vi "Dashboard Main.vi"() -> ()   [LabVIEW 2014]
uses:
  robot/Lightning base/Auton Modes.ctl
  <vilib>/event_ctls.llb/eventvkey.ctl
  VideoControlMode.ctl
  Video State.vi
  <vilib>/Rock Robotics/WPI/Dashboard/WPI_DashboardLogging Global.vi
  <vilib>/Utility/config.llb/Write Key (String).vi
  <vilib>/Utility/config.llb/Write Key (I32).vi
  <vilib>/Rock Robotics/Network Tables/SD Write Number.vi
  <vilib>/Utility/config.llb/NI_LVConfig.lvlib
panel:
  out "Video Mode":bool
  out "OpenIniState":enum16{"Waiting", "SwitchModeHappening"}(ring)
  out "Joystick":dbl
  out "POV[0]":dbl
  out "CameraSwitchModeState":enum16{"Waiting", "SwitchModeHappening"}(ring)
  out "Camera Mode":bool
  out "GetIniState":enum16{"Waiting", "SwitchModeHappening"}(ring)
  out "SetIniState":enum16{"Waiting", "SwitchModeHappening"}(ring)
  in  "TCP":refnum<k5>
  in  "Rec Mode":enum32{"Stop", "Record", "Playback"}(radio)
  in  "Vision":u16(ring) items=["Camera Off", "USB Camera SW", "USB Camera HW", "IP Camera"]
  out "Camera IP":string
  out "Image Message":string="Timeout in Camera Communications"
  in  "Dashboard Tab":T1(tab)=enum."Auton"
  in  "Camera Settings":T2={"Frame Rate"=30, "Compression"=30, "Size"=1} {"Frame Rate" scale=1.0..30.0; "Size" items=["640x480", "320x240", "160x120"]}
  out "MotorChart R":cluster{"Numeric":dbl, "Numeric":dbl}(graph)
  out "MotorChart L":T3(graph)
  out "MotorSliders R":cluster{"MotorSlide1":dbl, "MotorSlide2":dbl} {"MotorSlide2" scale=-1.0..1.0 scale format="%#_2e"; "MotorSlide1" scale=-1.0..1.0 scale format="%#_2e"}
  out "MotorSliders L":T4 {"MotorSlide4 2" scale=0.0..14.0 scale format="%#_2e"; "MotorSlide2" scale=-1.0..1.0 scale format="%#_2e"; "MotorSlide1" scale=-1.0..1.0 scale format="%#_2e"}
  out "Gyro":dbl(knob) scale=0.0..360.0
  out "JS1 Z":dbl(slide) scale=-1.0..1.0 scale format="%#_2e"
  out "JS1 Graph":cluster{"X":dbl, "Y":dbl}[](graph)
  out "JS1 Buttons":T5
  out "JS2 Z":dbl(slide) scale=-1.0..1.0 scale format="%#_2e"
  out "JS2 Graph":cluster{"X":dbl, "Y":dbl}[](graph)
  out "JS2 Buttons":T5
  out "Mode":T6(ring)=enum."Auto Disabled"
  in  "DB Camera Config":bool
  out "fps":dbl format="%#.1g"
  out "Mbps":dbl format="%#.1g"
  out "Mbps 2":bool
  in  "Camera Joystick Controller":enum16{"Joystick 1", "Joystick 2"}(ring)
  in  "Camera Choice":enum16{"Front", "Back"}(ring)
  in  "CG Drive Delay":dbl
  in  "CG Power2":dbl
  in  "CG Drive Distance":dbl
  in  "CG Power":dbl
  in  "CG Time2":dbl
  in  "CG Time":dbl
  in  "DriverAutonFile":string
  in  "CoPilotAutonFile":string
  in  "Auton Distance":dbl=2.0
  in  "Auton Mode":T7
  out "FTP Result":u32(colorbox)
  in  "Open INI File":bool
  in  "RoboRIO IP address":string="10.8.62.12"
  in  "Robot Full Path":string="/home/lvuser/calibrations/cals.ini"
  in  "Local Path":path=path "C:/FRC/Calibrations/cals.ini"
  in  "Send INI":bool
  in  "Get INI File":bool
  in  "Test Slider":dbl(slide) scale=0.0..100.0 scale format="%#_3g"
  in  "On/Off":bool caption="Solenoid"
  in  "Test Name":u16(ring) items=["Select the test to run...", "Example Test", "-------------------------------", "List of tests is built in robot code.", "Replace with your own automated tests."]
  in  "Test Tree":string(tree)
  in  "Motor":cluster{"Value":dbl, "Enable":bool} {"Value" scale=-1.0..1.0 scale format="%#_3g"}
  out "Progress":T8 {"Test Progress" scale=0.0..100.0}
  in  "Rev/Fwd":cluster{"Forward":bool, "Reverse":bool}
  in  "Test Ring":u16(ring) items=["Monochrome", "Color"]
  in  "Listbox":i32(listbox)
  out "Tree":string(tree)
  in  "PID":bool
  in  "DeadZone":dbl
  in  "PIDi":dbl
  in  "PIDd":dbl
  in  "Max Velocity":dbl
  in  "DriveRamp":dbl
  in  "PIDp":dbl
  in  "DriveSkew":dbl
  in  "MinMotorPower":dbl
  in  "MinJoystickChange":dbl
  in  "Drive Slice Time":dbl
  out "Camera Image":T9(plugin-control)
  out "Boolean":bool
  # "Left"
  # "Front"
  # "Right"
  # "Battery"
  # "Base file names, assumed to be\n/home/lvuser/auton"
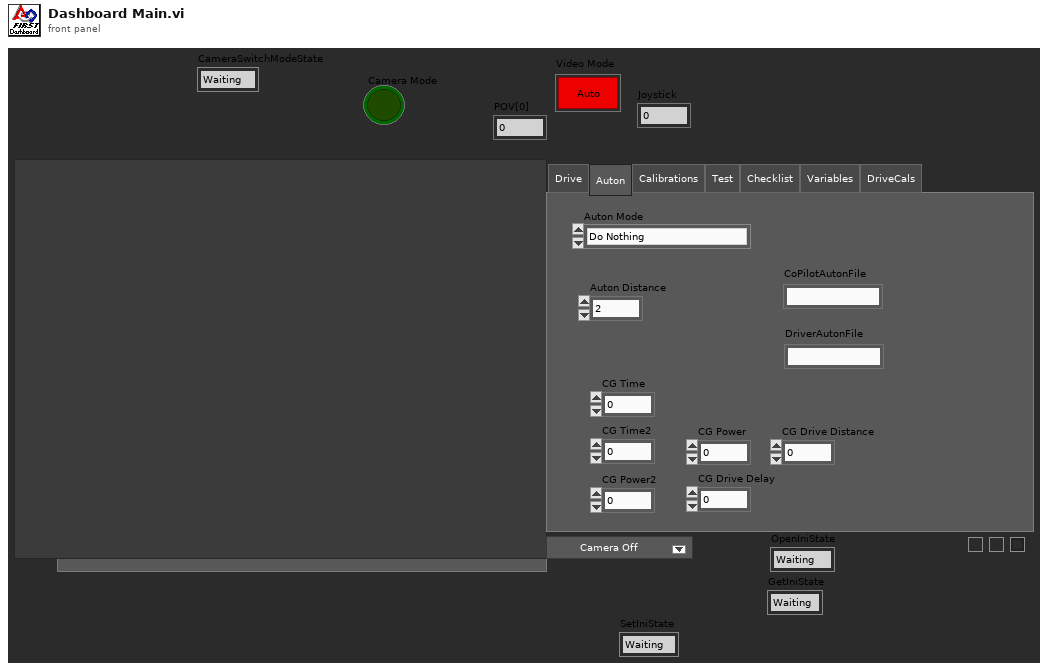
[diagram p1: front panel]
types:
  T1 = enum32{"Drive", "Auton", "Calibrations", "Test", "Checklist", "Variables", "DriveCals"}
  T2 = cluster{"Frame Rate":i32, "Compression":i32, "Size":u16}
  T3 = cluster{"Numeric":dbl, "Numeric":dbl, "Battery V":dbl}
  T4 = cluster{"MotorSlide1":dbl, "MotorSlide2":dbl, "MotorSlide4 2":dbl}
  T5 = cluster{bool, bool, bool, bool, bool, bool, bool, bool, bool, bool, bool, bool}
  T6 = enum8{"Tele-Op Disabled", "Tele-Op Enabled", "Auto Disabled", "Auto Enabled", "Test Disabled", "Test Enabled", "Disconnected", "No Code", "E-Stop"}
  T7 = typedef "Auton Modes.ctl" = enum16{"Do Nothing", "Snake", "Move Forward", "Move Forward w/Tote", "Move Forward w/RC", "Gather RC from Step", "3 Tote Auton", "Vision Test", "Strafer", "Pick up rc"}
  T8 = cluster{"Test Progress":u8, "Test Progress Text":string}
  T9 = typedef "IMAQ Image.ctl" = refnum<image>
  T10 = enum32{"Drive", "Basic", "Custom", "Test", "Checklist", "Variables", "DriveCals"}
  T11 = enum32{"Drive", "Basic", "Custom", "Test", "Checklist", "Variables"}
  T12 = enum32{"Drive", "Auton", "Custom", "Test", "Checklist", "Variables"}
  T13 = typedef "Image Type" = u32
  T14 = enum16{"Waiting", "SwitchModeHappening", "SwitchDone"}
  T15 = typedef "VideoControlMode.ctl" = enum16{"HatControl", "JoystickControl"}
  T16 = cluster{"Camera Image":refnum<vi>, "Dashboard Tab":refnum<vi>, "Boolean":refnum<vi>, "Vision":refnum<vi>, "Rec Mode":refnum<vi>, "Test Slider":refnum<vi>, "On/Off ":refnum<vi>, "Test Ring":refnum<vi>, "Rev/Fwd":refnum<vi>, "Test Name":refnum<vi>, "Motor":refnum<vi>, "Progress":refnum<vi>, "CheckList":refnum<vi>, "Tree":refnum<vi>, "Test Tree":refnum<vi>}
  T17 = cluster{"Desired Font (Application)":enum16{"User-specified Font", "Application Font", "System Font", "Dialog Font"}, "[User-specified Font]":cluster{"Font Name":string, "Size":i16, "Strikeout?":bool, "Italic?":bool, "Underline?":bool, "Outline?":bool, "Shadow?":bool, "Bold?":bool, "Rotation Angle":dbl}, "Horizontal Alignment":i16, "Vertical Alignment":i16}
  T18 = cluster{"Error Strings":string, "Disable Counts":cluster{u16, u16}, "Rail Faults":cluster{u16, u16, u16}, "Robot IP":string, "DB Mode":u8, "Event Info":cluster{"Name":string, "Type":u8, "Number":u16, "Replay":u8}, "Camera Addr":string}
  T19 = cluster{"Storage":cluster{"Disk Free":u64, "RAM Block":u32, "RAM free":u32}, "CPU Utilization":cluster{"CPU % ISR":sgl, "CPU % Time Crit":sgl, "CPU % Timed Str":sgl, "CPU % High":sgl, "CPU % Above":sgl, "CPU % Normal":sgl, "CPU % Low":sgl}, "CAN":cluster{"% Bus Utilization":sgl, "Bus Off Cnt":u32, "TX_FIFO Full Cnt":u32, "Receive Error Cnt":u8, "Transmit Error Cnt":u8}, "HID":cluster{"HID Outputs":u32, "Rumble Low":u16, "Rumble High":u16}[]}
  T20 = cluster{"Status bits":cluster{"Test Mode":bool, "Autonomous":bool, "Enabled":bool, "Code Start":bool, "Brownout":bool, "Reserved 2":bool, "Reserved 3":bool, "E-Stop":bool}, "Code Trace":cluster{"Disabled":bool, "TeleOp":bool, "Auto":bool, "Test":bool}, "Controller Type":enum16{"unknown", "cRIO", "roboRio"}, "Code?":enum16{"unknown", "noCode", "code"}, "Battery V":dbl}
  T21 = cluster{"Control Bits":cluster{"TestMode":bool, "Autonomous":bool, "Enabled":bool, "FMS Present":bool, bool, bool, bool, "E-Stop":bool}, "Team Station ":u8, "Countdown":sgl, "Joystick Values":cluster{"Axes":dbl[], "Buttons":bool[], "POVs":i16[]}[]}
  T22 = cluster{"Axes":dbl[], "Buttons":bool[], "POVs":i16[]}[]
  T23 = cluster{"Disabled":bool, "TeleOp":bool, "Auto":bool, "Test":bool}
  T24 = cluster{"Axes":dbl[], "Buttons":bool[], "POVs":i16[]}
  T25 = cluster{"Buttons[0]":bool, "Buttons[1]":bool, "Buttons[2]":bool, "Buttons[3]":bool, "Buttons[4]":bool, "Buttons[5]":bool, "Buttons[6]":bool, "Buttons[7]":bool, "Buttons[8]":bool}
  T26 = cluster{"POVs[0]":i16, "POVs[1]":i16, "POVs[2]":i16, "POVs[3]":i16, "POVs[4]":i16, "POVs[5]":i16, "POVs[6]":i16, "POVs[7]":i16, "POVs[8]":i16}
  T27 = cluster{"Axes[0]":dbl, "Axes[1]":dbl, "Axes[2]":dbl, "Axes[3]":dbl, "Axes[4]":dbl, "Axes[5]":dbl, "Axes[6]":dbl, "Axes[7]":dbl, "Axes[8]":dbl}
  T28 = cluster{"Buttons[0]":bool, "Buttons[1]":bool, "Buttons[2]":bool, "Buttons[3]":bool, "Buttons[4]":bool, "Buttons[5]":bool, "Buttons[6]":bool, "Buttons[7]":bool, "Buttons[8]":bool, "Buttons[9]":bool, "Buttons[10]":bool, "Buttons[11]":bool}
  T29 = typedef "NI_LVConfig.lvlib/Config Data RefNum.ctl" = refnum<k1>
  T30 = cluster{"Operation":enum16{"Update", "Clear"}, "Color Box":u32}[]
  T31 = typedef "eventvkey.ctl" = enum16{"ASCII", "Enter", "Return", "Shift", "Ctrl", "Alt", "Cmd", "Opt", "Caps", "NumLock", "Clear", "Break", "Up", "Down", "Left", "Right", "Insert", "Delete", "Home", "End", "PageUp", "PageDown", "Escape", "Help", "Pause", "ScrollLock", "F1", "F2", "F3", "F4", "F5", "F6", "F7", "F8", "F9", "F10", "F11", "F12", "F13", "F14", "F15", "F16", "F17", "F18", "F19", "F20", "F21", "F22", "F23", "F24", "Play", "VolumeUp", "VolumeDown", "Mute", "Two Byte Char"}
  T32 = cluster{"Image Size":bool, "Image Type":bool, "Pixel Value":bool, "ROI Information":bool, "Zoom Factor":bool}
  T33 = enum8{"Enabled", "Disabled", "Disabled and Grayed Out"}
  T34 = cluster{"Operation":enum16{"Update", "Clear"}, "Color Box":u32}
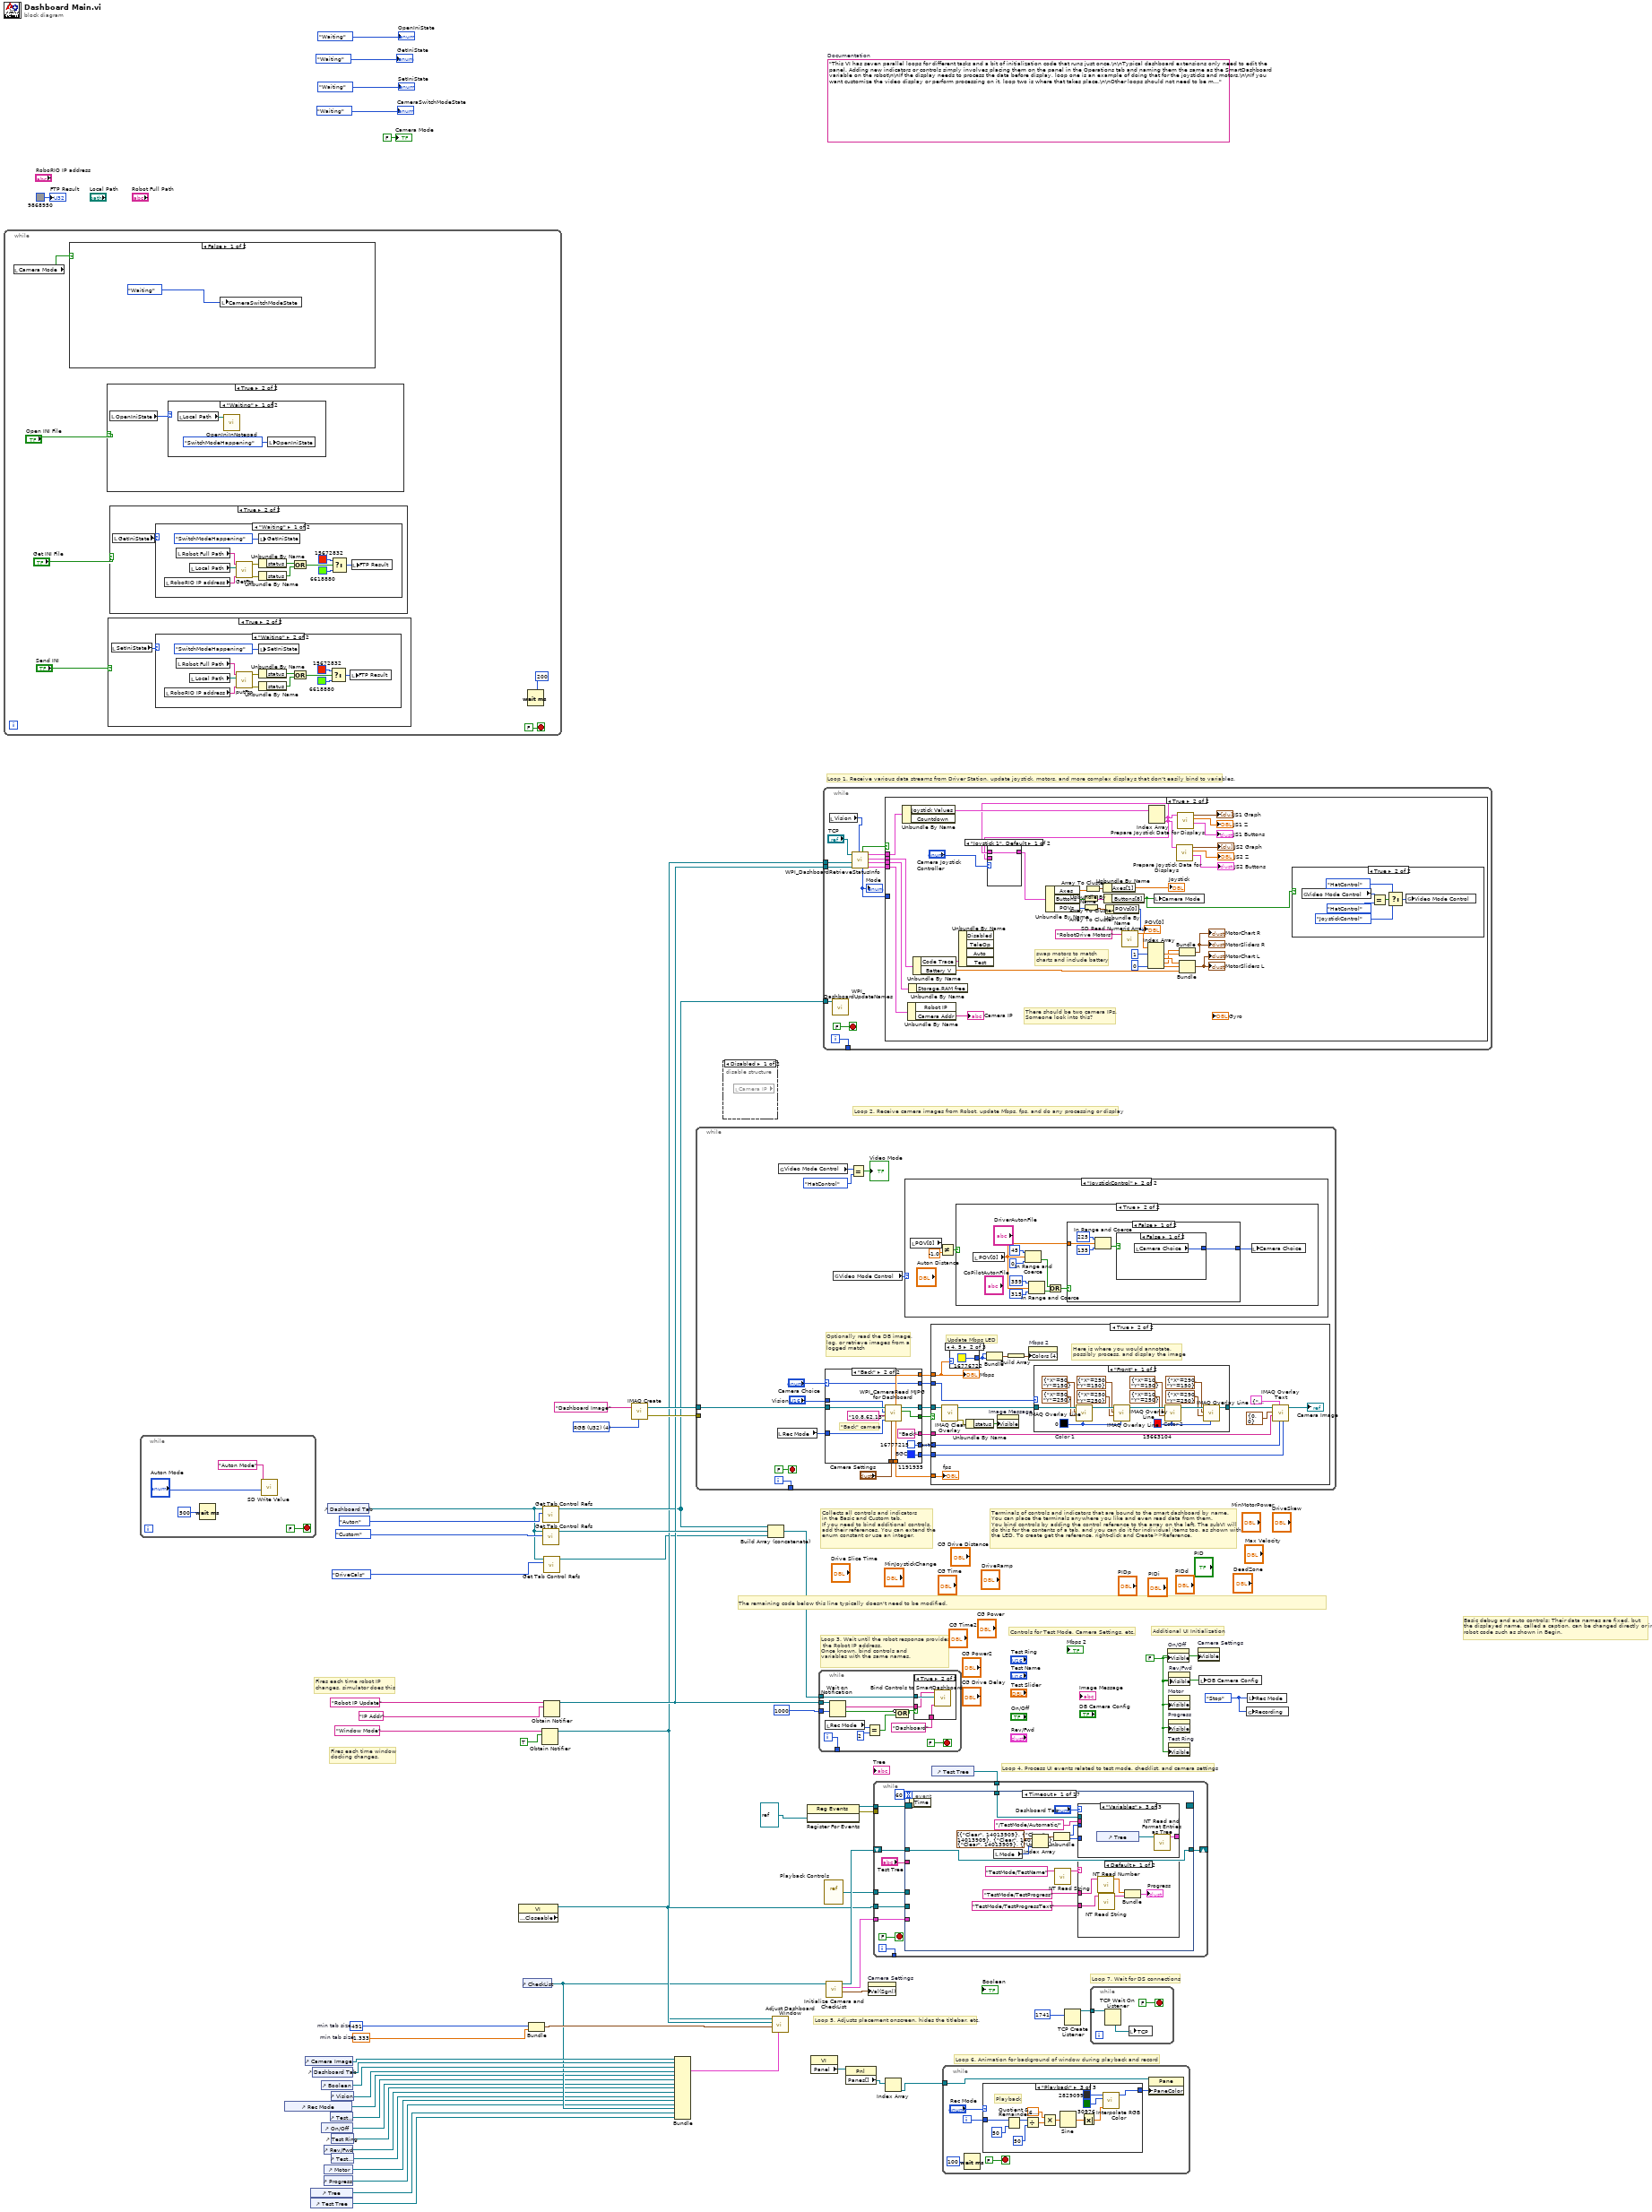
[diagram p0: block diagram]
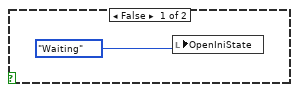
[diagram p3: hidden frame]
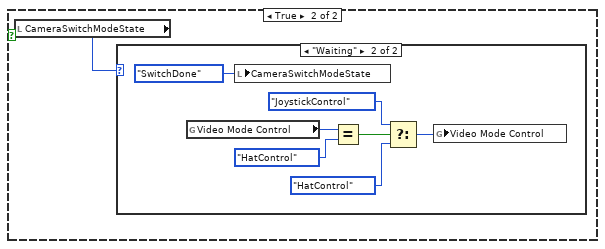
[diagram p5: hidden frame]
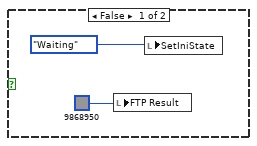
[diagram p7: hidden frame]
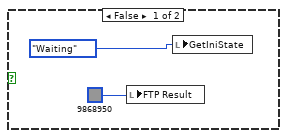
[diagram p9: hidden frame]
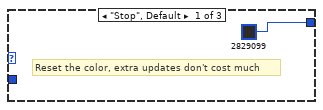
[diagram p14: hidden frame]
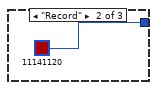
[diagram p15: hidden frame]
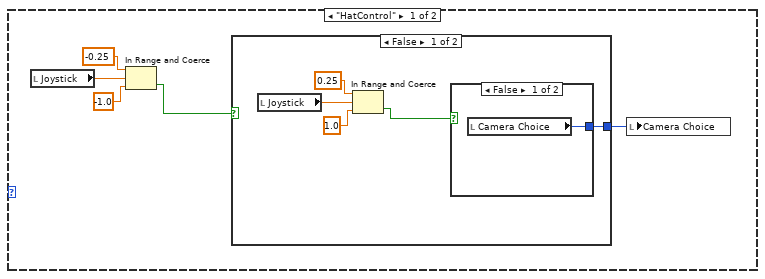
[diagram p17: hidden frame]
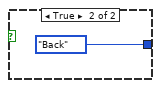
[diagram p18: hidden frame]
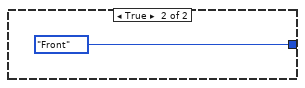
[diagram p19: hidden frame]
diagram:
  w33 = 491  # min tab size
  w32 = 1.333  # min tab size
  w40 = enum32{"Stop", "Record", "Playback"}."Stop" ("Rec Mode")
  w15 = FALSE ("Visible")
  (unwired) "This VI has seven parallel loops for different tasks and a bit of initialization code that runs just once.\n\nTypical dashboard extensions only need to edit the panel. Adding new indicators or controls simply involves placing them on the panel in the Operations tab and naming them the same as the SmartDashboard variable on the robot\n\nIf the display needs to process the data before display, loop one is an example of doing that for the joysticks and motors.\n\nIf you want customize the video display or perform processing on it, loop two is where that takes place.\n\nOther loops should not need to be modified. They are pretty standard, and document the task they perform."  # Documentation
  w60 = T13 4 items=["Grayscale (U8)", "Grayscale (I16)", "Grayscale (SGL)", "Complex (CSG)", "RGB (U32)", "HSL (U32)", "RGB (U64)"] ("Image Type")
  # "Loop 7. Wait for DS connections"
  # "Basic debug and auto controls: Their data names are fixed, but\nthe displayed name, called a caption, can be changed directly or in\nrobot code such as shown in Begin."
  # "Controls for Test Mode, Camera Settings, etc."
  # "Additional UI Initialization"
  # "Loop 6. Animation for background of window during playback and record"
  # "Fires each time robot IP\nchanges, simulator does this"
  # "Fires each time window\ndocking changes."
  # "Collects all controls and indicators\nin the Basic and Custom tab.\nIf you need to bind additional controls,\nadd their references. You can extend the\nenum constant or use an integer."
  # "The remaining code below this line typically doesn't need to be modified."
  # "Loop 4. Process UI events related to test mode, checklist, and camera settings"
  # "Terminals of controls and indicators that are bound to the smart dashboard by name.\nYou can place the terminals anywhere you like and even read data from them.\nYou bind controls by adding the control reference to the array on the left. The subVI will\ndo this for the contents of a tab, and you can do it for individual items too, as shown with\nthe LED. To create get the reference, right-click and Create>>Reference."
  # "Loop 3. Wait until the robot response provides\n the Robot IP address.\nOnce known, bind controls and\nvariables with the same names."
  # "Loop 5. Adjusts placement onscreen, hides the titlebar, etc."
  # "Loop 1. Receive various data streams from Driver Station, update joystick, motors, and more complex displays that don't easily bind to variables."
  # "Loop 2. Receive camera images from Robot, update Mbps, fps, and do any processing or display"
  n1 = while {
    stop <- FALSE stop-if-true
    n2 = local read "Camera Mode"() -> (w62:bool)
    n3 = case shown="False" w62 {
      frame False {
        n4 = local write "CameraSwitchModeState"(T14."Waiting" ("CameraSwitchMode")) -> ()
      }
      frame True {
        n5 = local read "CameraSwitchModeState"() -> (w72:enum16{"Waiting", "SwitchModeHappening"})
        n6 = case shown="\"Waiting\"" w72 {
          frame "SwitchModeHappening" {
          }
          frame "Waiting" {
            n7 = global read "Video State.vi" "Video Mode Control"() -> (w75:enum16{"HatControl", "JoystickControl"})
            n8 = local write "CameraSwitchModeState"(T14."SwitchDone" ("CameraSwitchMode")) -> ()
            n9 = Equal?(x=w75, y=enum16{"HatControl", "JoystickControl"}."HatControl" ("f")) -> (x = y?=w76:bool)
            n10 = Select(t=VideoControlMode."JoystickControl" ("f"), s=w76, f=enum16{"HatControl", "JoystickControl"}."HatControl") -> (s? t:f=w77:T15)
            n11 = global write "Video State.vi" "Video Mode Control"(w77) -> ()
          }
        }
      }
    }
    n12 = case shown="True" "Open INI File" {
      frame False {
        n13 = local write "OpenIniState"(T14."Waiting" ("GetIniState")) -> ()
      }
      frame True {
        n14 = local read "OpenIniState"() -> (w68:enum16{"Waiting", "SwitchModeHappening"})
        n15 = case shown="\"Waiting\"" w68 {
          frame "Waiting" {
            n16 = local read "Local Path"() -> (w69:path)
            n17 = call "OpenIniInNotepad.vi"("Path"=w69) -> ()  [unwired: 11 in]
            n18 = local write "OpenIniState"(T14."SwitchModeHappening" ("SetIniState")) -> ()
          }
          frame "SwitchModeHappening" {
          }
        }
      }
    }
    n19 = case shown="True" "Send INI" {
      frame False {
        n20 = local write "FTP Result"(u32 9868950 ("Color Box")) -> ()
        n21 = local write "SetIniState"(T14."Waiting" ("SetIniState")) -> ()
      }
      frame True {
        n22 = local read "SetIniState"() -> (w82:enum16{"Waiting", "SwitchModeHappening"})
        n23 = case shown="\"Waiting\"" w82 {
          frame "SwitchModeHappening" {
          }
          frame "Waiting" {
            n24 = local read "RoboRIO IP address"() -> (w93:string)
            n25 = local read "Robot Full Path"() -> (w92:string)
            n26 = local read "Local Path"() -> (w91:path)
            n27 = call "putFtp.vi"("host"=w93, "local path"=w91, "remote path"=w92) -> ("file error out"=w83:errorcluster, "ftp error out 2"=w84:errorcluster)  [unwired: 7 in]
            n28 = local write "SetIniState"(T14."SwitchModeHappening" ("SetIniState")) -> ()
            n29 = Unbundle By Name(w84) -> ("status"=w85:bool)
            n30 = Unbundle By Name(w83) -> ("status"=w86:bool)
            n31 = Or(x=w85, y=w86) -> (x .or. y?=w87:bool)
            n32 = Select(t=u32 15672832 ("Color Box"), s=w87, f=u32 6618880 ("Color Box")) -> (s? t:f=w88:u32)
            n33 = local write "FTP Result"(w88) -> ()
          }
        }
      }
    }
    n34 = case shown="True" "Get INI File" {
      frame False {
        n35 = local write "FTP Result"(u32 9868950 ("Color Box")) -> ()
        n36 = local write "GetIniState"(T14."Waiting" ("GetIniState")) -> ()
      }
      frame True {
        n37 = local read "GetIniState"() -> (w97:enum16{"Waiting", "SwitchModeHappening"})
        n38 = case shown="\"Waiting\"" w97 {
          frame "Waiting" {
            n39 = local read "RoboRIO IP address"() -> (w108:string)
            n40 = local read "Robot Full Path"() -> (w106:string)
            n41 = local read "Local Path"() -> (w107:path)
            n42 = call "GetFtp.vi"("host"=w108, "local path"=w107, "remote path"=w106) -> ("file error out"=w104:errorcluster, "ftp error out 2"=w105:errorcluster)  [unwired: 7 in]
            n43 = local write "GetIniState"(T14."SwitchModeHappening" ("SetIniState")) -> ()
            n44 = Unbundle By Name(w105) -> ("status"=w103:bool)
            n45 = Unbundle By Name(w104) -> ("status"=w102:bool)
            n46 = Or(x=w103, y=w102) -> (x .or. y?=w101:bool)
            n47 = Select(t=u32 15672832 ("Color Box"), s=w101, f=u32 6618880 ("Color Box")) -> (s? t:f=w100:u32)
            n48 = local write "FTP Result"(w100) -> ()
          }
          frame "SwitchModeHappening" {
          }
        }
      }
    }
    n49 = Wait (ms)(milliseconds to wait=u32 200) -> ()  [unwired: 1 out]
  }
  n50 = while {
    stop <- FALSE stop-if-true
    n51 = Wait (ms)(milliseconds to wait=u32 500) -> ()  [unwired: 1 out]
    n52 = call-poly <vilib>:"SD Write Value.vi"("Numeric"="Auton Mode", "Name"="Auton Mode") -> ()  [unwired: 8 in, 2 out]
  }
  n53 = control-ref of="Rec Mode"() -> (w21:refnum<vi>)
  n54 = control-ref of="Camera Image"() -> (w36:refnum<vi>)
  n55 = control-ref of="Tree"() -> (w25:refnum<vi>)
  n56 = control-ref of="Test Tree"() -> (w24:refnum<vi>)
  n57 = control-ref of="Dashboard Tab"() -> (w35:refnum<vi>)
  n58 = control-ref of="Boolean"() -> (w30:refnum<vi>)
  n59 = control-ref of="On/Off"() -> (w19:refnum<vi>)
  n60 = control-ref of="Progress"() -> (w16:refnum<vi>)
  n61 = control-ref of="Rev/Fwd"() -> (w17:refnum<vi>)
  n62 = control-ref of="Motor"() -> (w22:refnum<vi>)
  n63 = control-ref of="Dashboard Tab"() -> (w8:refnum<vi>)
  n64 = control-ref of="Test Slider"() -> (w20:refnum<vi>)
  n65 = control-ref of="Vision"() -> (w34:refnum<vi>)
  n66 = control-ref of="Test Ring"() -> (w18:refnum<vi>)
  n67 = control-ref of="Test Name"() -> (w23:refnum<vi>)
  n68 = property class="VI" props=["Front Panel.Closeable"]() -> (reference out=w39:refnum<vi>)  [unwired: 2 in, 2 out]
  n69 = control-ref of="CheckList"() -> (w26:refnum<vi>)
  n70 = Bundle("min tab size"=w33, "min tab size"=w32) -> (w31:cluster{"min tab size":i32, "min tab size":dbl})  [unwired: 1 in]
  n71 = Obtain Notifier(name (unnamed)="Window Mode", notification data type=TRUE) -> (notifier out=w12:refnum<notifier>)  [unwired: 2 in, 2 out]
  n72 = call <vilib>:"Get Tab Control Refs.vi"("Page Index"=T12."Auton" ("Dashboard Tab"), "TabControl in"=w8) -> ("ControlsOnPage"=w13:refnum<vi>[])  [unwired: 9 in]
  n73 = call <vilib>:"Get Tab Control Refs.vi"("Page Index"=T11."Custom" ("Dashboard Tab"), "TabControl in"=w8) -> ("ControlsOnPage"=w38:refnum<vi>[])  [unwired: 9 in]
  n74 = call <vilib>:"Get Tab Control Refs.vi"("Page Index"=T10."DriveCals" ("Dashboard Tab"), "TabControl in"=w8) -> ("ControlsOnPage"=w7:refnum<vi>[])  [unwired: 9 in]
  n75 = Obtain Notifier(name (unnamed)="Robot IP Update", notification data type="IP Addr" ("name (unnamed)")) -> (notifier out=w14:refnum<notifier>)  [unwired: 2 in, 2 out]
  n76 = call "IMAQ Create"("Image Name"="Dashboard Image", "Image Type"=w60) -> ("New Image"=w58:T9, "error out"=w57:errorcluster)  [unwired: 2 in, 1 out]
  n77 = Bundle("Camera Image"=w36, "Dashboard Tab"=w35, "Boolean"=w30, "Vision"=w34, "Rec Mode"=w21, "Test Slider"=w20, "On/Off"=w19, "Test Ring"=w18, "Rev/Fwd"=w17, "Test Name"=w23, "Motor"=w22, "Progress"=w16, "CheckList"=w26, "Tree"=w25, "Test Tree"=w24) -> (w27:T16)  [unwired: 1 in]
  n78 = while {
    tunnel: w58 -> [w130]
    tunnel: w57 -> [_]
    tunnel: [w131] -> _
    i -> [w131]
    stop <- FALSE stop-if-true
    # "Optionally read the DB image,\nlog, or retrieve images from a\nlogged match"
    n79 = local read "Rec Mode"() -> (w124:enum32{"Stop", "Record", "Playback"})
    n80 = global read "Video State.vi" "Video Mode Control"() -> (w114:enum16{"HatControl", "JoystickControl"})
    n81 = case shown="\"Back\"" "Camera Choice" {
      selector: "Camera Choice" -> [w166 w179]
      tunnel: w130 -> [w178 w191]
      tunnel: [w177 w190] -> w129
      tunnel: [w176 w189] -> w128
      tunnel: [w175 w188] -> w127
      tunnel: [w174 w187] -> w126
      tunnel: "Camera Settings" -> [w173 w186]
      tunnel: w124 -> [w172 w185]
      tunnel: "Vision" -> [w170 w183]
      tunnel: ["Front" "Back"] -> w121
      tunnel: [w167 w181] -> w120
      tunnel: [w168 w180] -> w119
      tunnel: [w166 w179] -> w118
      frame "Front" {
        w168 = u32 0  # TextC
        w167 = u32 16743698  # BGC
        # "\"Front\" camera"
        n82 = call <vilib>:"WPI_CameraRead MJPG for Dashboard.vi"("Camera Settings"=w173, "Rec Mode"=w172, "Camera IP"="10.8.62.11", "Camera Mode"=w170, "Refnum in"=w178) -> ("Active"=w176:bool, "Refnum out"=w177:T9, "FPS"=w175:dbl, "Bandwidth (Mbps)"=w174:dbl)  [unwired: 3 in]
      }
      frame "Back" {
        w180 = u32 16777215  # TextC
        w181 = u32 1191935  # BGC
        # "\"Back\" camera"
        n83 = call <vilib>:"WPI_CameraRead MJPG for Dashboard.vi"("Camera Settings"=w186, "Rec Mode"=w185, "Camera IP"="10.8.62.13", "Camera Mode"=w183, "Refnum in"=w191) -> ("Active"=w189:bool, "Refnum out"=w190:T9, "FPS"=w188:dbl, "Bandwidth (Mbps)"=w187:dbl)  [unwired: 3 in]
      }
    }
    n84 = global read "Video State.vi" "Video Mode Control"() -> (w117:enum16{"HatControl", "JoystickControl"})
    n85 = Equal?(x=w114, y=enum16{"HatControl", "JoystickControl"}."HatControl") -> (x = y?=→"Video Mode":bool)
    n86 = case shown="\"JoystickControl\"" w117 {
      frame "HatControl" {
        n87 = local read "Joystick"() -> (w136:dbl)
        n88 = In Range and Coerce(upper limit=-0.25, x=w136, lower limit=-1.0) -> (In Range?=w135:bool)  [unwired: 1 out]
        n89 = case shown="False" w135 {
          tunnel: [w142 enum16{"Front", "Back"}."Front" ("Camera Choice 2")] -> w137
          frame False {
            n90 = local read "Joystick"() -> (w139:dbl)
            n91 = In Range and Coerce(upper limit=0.25, x=w139, lower limit=1.0) -> (In Range?=w138:bool)  [unwired: 1 out]
            n92 = case shown="False" w138 {
              tunnel: [w143 enum16{"Front", "Back"}."Back" ("Camera Choice 2")] -> w142
              frame False {
                n93 = local read "Camera Choice"() -> (w143:enum16{"Front", "Back"})
              }
              frame True {
              }
            }
          }
          frame True {
          }
        }
        n94 = local write "Camera Choice"(w137) -> ()
      }
      frame "JoystickControl" {
        n95 = local read "POV[0]"() -> (w146:dbl)
        n96 = Not Equal?(x=w146, y=-1.0) -> (x != y?=w148:bool)
        n97 = case shown="True" w148 {
          frame False {
          }
          frame True {
            n98 = local read "POV[0]"() -> (w153:dbl)
            n99 = In Range and Coerce(upper limit=i16 45 ("y"), x=w153, lower limit=i16 0 ("y")) -> (In Range?=w156:bool)  [unwired: 1 out]
            n100 = In Range and Coerce(upper limit=i16 359 ("y"), x=w153, lower limit=i16 315 ("y")) -> (In Range?=w150:bool)  [unwired: 1 out]
            n101 = Or(x=w156, y=w150) -> (x .or. y?=w157:bool)
            n102 = case shown="False" w157 {
              tunnel: w153 -> [w160 _]
              tunnel: [w158 enum16{"Front", "Back"}."Front" ("Camera Choice 2")] -> w149
              frame False {
                n103 = In Range and Coerce(upper limit=i16 225 ("y"), x=w160, lower limit=i16 135 ("y")) -> (In Range?=w159:bool)  [unwired: 1 out]
                n104 = case shown="False" w159 {
                  tunnel: [w163 enum16{"Front", "Back"}."Back" ("Camera Choice 2")] -> w158
                  frame False {
                    n105 = local read "Camera Choice"() -> (w163:enum16{"Front", "Back"})
                  }
                  frame True {
                  }
                }
              }
              frame True {
              }
            }
            n106 = local write "Camera Choice"(w149) -> ()
          }
        }
      }
    }
    n107 = case shown="True" w128 {
      tunnel: w129 -> [_ w204]
      tunnel: w126 -> [_ w203]
      tunnel: w127 -> [_ w202]
      tunnel: w121 -> [_ w197]
      tunnel: w120 -> [_ w198]
      tunnel: w119 -> [_ w194]
      tunnel: w118 -> [_ w193]
      frame False {
        # "Sleep for 500ms"
        n108 = Wait Until Next ms Multiple(millisecond multiple=u32 500) -> ()  [unwired: 1 out]
      }
      frame True {
        # "Here is where you would annotate,\npossibly process, and display the image"
        # "Update Mbps LED"
        n109 = call "IMAQ Clear Overlay"("Image"=w204) -> ("error out"=w208:errorcluster, "Image Out"=w196:T9)  [unwired: 2 in, 7 out]
        n110 = case shown="4, 5" w203 {
          tunnel: [u32 6618880 ("Color Box") u32 16776722 ("Color Box") u32 16716800 ("Color Box")] -> w205
          frame Default {
          }
          frame 4, 5 {
          }
          frame 6.. {
          }
        }
        n111 = Unbundle By Name(w208) -> ("status"=w209:bool)
        n112 = Bundle("Color Box"=w205, "Color Box"=w205) -> (w207:cluster{"Color Box":u32, "Color Box":u32})  [unwired: 1 out]
        n113 = property on="Image Message" class="Str"("Visible"=w209) -> ()  [unwired: 2 in, 2 out]
        n114 = Build Array(w207) -> (w206:cluster{"Color Box":u32, "Color Box":u32}[])
        n115 = property on="Mbps 2" class="Bool (strict)"("Colors [4]"=w206) -> ()  [unwired: 2 in, 2 out]
        n116 = case shown="\"Front\"" w193 {
          tunnel: w196 -> [w224 w225]
          tunnel: [w218 w225] -> w195
          frame "Front" {
            w217 = u32 15663104  # Color 2
            w221 = u32 0  # Color 1
            n117 = call "IMAQ Overlay Line"("Color"=w221, "End Point"=cluster{"X":i32, "Y":i32} {"X"=50, "Y"=250} ("Start Point"), "Start Point"=cluster{"X":i32, "Y":i32} {"X"=50, "Y"=150}, "Image"=w224) -> ("Image Out"=w222:T9)  [unwired: 6 in, 1 out]
            n118 = call "IMAQ Overlay Line"("Color"=w221, "End Point"=cluster{"X":i32, "Y":i32} {"X"=250, "Y"=250} ("Start Point"), "Start Point"=cluster{"X":i32, "Y":i32} {"X"=250, "Y"=150}, "Image"=w222) -> ("Image Out"=w220:T9)  [unwired: 6 in, 1 out]
            n119 = call "IMAQ Overlay Line"("Color"=w217, "End Point"=cluster{"X":i32, "Y":i32} {"X"=10, "Y"=250} ("Start Point"), "Start Point"=cluster{"X":i32, "Y":i32} {"X"=10, "Y"=150}, "Image"=w220) -> ("Image Out"=w219:T9)  [unwired: 6 in, 1 out]
            n120 = call "IMAQ Overlay Line"("Color"=w217, "End Point"=cluster{"X":i32, "Y":i32} {"X"=290, "Y"=250} ("Start Point"), "Start Point"=cluster{"X":i32, "Y":i32} {"X"=290, "Y"=150}, "Image"=w219) -> ("Image Out"=w218:T9)  [unwired: 6 in, 1 out]
          }
          frame "Back", Default {
          }
        }
        n121 = call "IMAQ Overlay Text"("BG Color (Transparent)"=w198, "Text Color (black)"=w194, "Font, Size & Style"=T17 {"Desired Font (Application)"=enum."User-specified Font", "[User-specified Font]"={"Font Name"="Comic Sans MS", "Size"=30, "Strikeout?"=FALSE, "Italic?"=FALSE, "Underline?"=TRUE, "Outline?"=TRUE, "Shadow?"=TRUE, "Bold?"=TRUE, "Rotation Angle"=0.0}, "Horizontal Alignment"=0, "Vertical Alignment"=1}, "String"=w197, "Origin"=cluster{"X":i32, "Y":i32} {"X"=0, "Y"=0}, "Image"=w195) -> ("Image Out"=→"Camera Image":T9)  [unwired: 4 in, 1 out]
        "Mbps" <- w203
        "fps" <- w202
      }
    }
  }
  n122 = disable-structure shown="Disabled" {
    frame Disabled {
      n123 = local read "Camera IP"() -> ()  [unwired: 1 out]
    }
    frame Enabled {
    }
  }
  n124 = Build Array (concatenate)(w13, w38, w7) -> (w37:refnum<vi>[])
  n125 = call "Adjust Dashboard Window.vi"("Sizing Refnums"=w27, "Size Constraints"=w31, "VI"=w39, "Notifier in"=w12) -> ()  [unwired: 8 in]
  n126 = register-events(refnum<vi> refnum) -> (reference out=w44:refnum<event-registration>, error out=w43:errorcluster)  [unwired: 2 in]
  n127 = property class="VI"() -> ("Panel"=w47:refnum<vi>)  [unwired: 2 in, 2 out]
  n128 = while {
    tunnel: w37 -> [w240]
    tunnel: w14 -> [w238]
    tunnel: [w236] -> _
    tunnel: u32 1000 ("milliseconds to wait") -> [w235]
    i -> [w236]
    stop <- FALSE stop-if-true
    n129 = local read "Rec Mode"() -> (w231:enum32{"Stop", "Record", "Playback"})
    n130 = Wait on Notification(notifier=w238, timeout in ms (-1)=w235) -> (notification=w237:string, timed out?=w233:bool)  [unwired: 2 in, 2 out]
    n131 = Equal?(x=w231, y=u16 2 ("Rec Mode")) -> (x = y?=w232:bool)
    n132 = Compound Arithmetic op=OR(invert w233, w232) -> (w234:bool)
    n133 = case shown="True" w234 {
      tunnel: w240 -> [_ w243]
      tunnel: w237 -> [_ w242]
      tunnel: "Dashboard" -> [_ w241]
      frame False {
      }
      frame True {
        n134 = call <vilib>:"Bind Controls to SmartDashboard.vi"("Client Name"=w241, "Bound Control Refs"=w243, "Server IP Address"=w242) -> ()  [unwired: 9 in]
      }
    }
  }
  n135 = while {
    tunnel: [w255] -> _
    tunnel: w14 -> [w249]
    tunnel: w13 -> [w248]
    tunnel: w12 -> [w244]
    i -> [w255]
    stop <- FALSE stop-if-true
    n136 = local read "Vision"() -> (w246:u16)
    n137 = call <vilib>:"WPI_DashboardUpdateNames.vi"("Controls on Tab"=w248) -> ()  [unwired: 11 in]
    n138 = call <vilib>:"WPI_DashboardRetrieveStatusInfo.vi"("Vision"=w246, "Binding Refnum"=w249, "Window Mode Notifier"=w244, "TCP Cnx"="TCP") -> ("Power and Errors"=w250:T18, "Robot Metrics"=w253:T19, "Status Info"=w254:T20, "Control Info"=w251:T21, "Robot Mode"=w247:T6, "Process?"=w252:bool)  [unwired: 2 in]
    "Mode" <- w247
    n139 = case shown="True" w252 {
      tunnel: w254 -> [_ w293]
      tunnel: w253 -> [_ w292]
      tunnel: w251 -> [_ w291]
      tunnel: w250 -> [_ w290]
      tunnel: w247 -> [_ _]
      frame False {
      }
      frame True {
        # "There should be two camera IPs.\nSomeone look into this?"
        # "swap motors to match\ncharts and include battery"
        n140 = Unbundle By Name(w291) -> ("Joystick Values"=w278:T22)  [unwired: 1 out]
        n141 = Unbundle By Name(w290) -> ("Camera Addr"=→"Camera IP":string)  [unwired: 1 out]
        n142 = Unbundle By Name(w292) -> ()  [unwired: 1 out]
        n143 = Unbundle By Name(w293) -> ("Code Trace"=w270:T23, "Battery V"=w279:dbl)
        n144 = Unbundle By Name(w270) -> ()  [unwired: 4 out]
        n145 = call <vilib>:"SD Read Numeric Array.vi"("Name"="RobotDrive Motors") -> ("Numeric Array"=w281:dbl[])  [unwired: 8 in, 2 out]
        n146 = Index Array(array=w281, index #1=1, index #4=0) -> (element #1=w285:dbl, element #2=w286:dbl, element #3=w284:dbl, element #4=w289:dbl)  [unwired: 2 in]
        n147 = Index Array(array=w278) -> (element #1=w260:T24, element #2=w259:T24)  [unwired: 2 in]
        n148 = case shown="\"Joystick 1\", Default" "Camera Joystick Controller" {
          tunnel: w260 -> [w300 _]
          tunnel: [w300 w301] -> w258
          tunnel: w259 -> [_ w301]
          frame "Joystick 1", Default {
          }
          frame "Joystick 2" {
          }
        }
        n149 = Unbundle By Name(w258) -> ("Axes"=w265:dbl[], "Buttons"=w267:bool[], "POVs"=w269:i16[])
        n150 = Array To Cluster(array=w267) -> (cluster=w266:T25)
        n151 = Array To Cluster(array=w269) -> (cluster=w268:T26)
        n152 = Array To Cluster(array=w265) -> (cluster=w264:T27)
        n153 = Unbundle By Name(w264) -> ("Axes[1]"=→"Joystick":dbl)
        n154 = Unbundle By Name(w266) -> ("Buttons[8]"=w257:bool)
        n155 = Unbundle By Name(w268) -> ("POVs[0]"=→"POV[0]":i16)
        n156 = local write "Camera Mode"(w257) -> ()
        n157 = call "Prepare Joystick Data for Displays.vi"("Joystick Values"=w259) -> ("Buttons"=→"JS2 Buttons":T28, "Z Axis"=→"JS2 Z":dbl, "Cartesian Data"=→"JS2 Graph":cluster{"X axis":dbl, "X axis":dbl}[])  [unwired: 8 in]
        n158 = call "Prepare Joystick Data for Displays.vi"("Joystick Values"=w260) -> ("Buttons"=→"JS1 Buttons":T28, "Z Axis"=→"JS1 Z":dbl, "Cartesian Data"=→"JS1 Graph":cluster{"X axis":dbl, "X axis":dbl}[])  [unwired: 8 in]
        n159 = Bundle("Numeric"=w284, "Numeric"=w285) -> (→"MotorChart R" →"MotorSliders R":cluster{"Numeric":dbl, "Numeric":dbl})  [unwired: 1 in]
        n160 = Bundle("Numeric"=w286, "Numeric"=w289, "Battery V"=w279) -> (→"MotorChart L" →"MotorSliders L":T3)  [unwired: 1 in]
        n161 = case shown="True" w257 {
          frame False {
          }
          frame True {
            n162 = global read "Video State.vi" "Video Mode Control"() -> (w295:enum16{"HatControl", "JoystickControl"})
            n163 = Equal?(x=w295, y=enum16{"HatControl", "JoystickControl"}."HatControl" ("f")) -> (x = y?=w296:bool)
            n164 = Select(t=enum16{"HatControl", "JoystickControl"}."HatControl" ("f"), s=w296, f=enum16{"HatControl", "JoystickControl"}."JoystickControl") -> (s? t:f=w297:enum16{"HatControl", "JoystickControl"})
            n165 = global write "Video State.vi" "Video Mode Control"(w297) -> ()
          }
        }
      }
    }
  }
  n166 = vi-ref "Playback Controls.vi"() -> (w45:refnum<vi>)
  n167 = call "Initialize Camera and CheckList.vi"("ListBox in"=w26) -> ("Cluster"=w51:cluster{"value":i32, "value":i32, "index":i32}, "Array"=w52:cluster{string[]}[], "File Refnum"=w50:T29)  [unwired: 8 in]
  n168 = property class="Pnl"(reference=w47) -> ("Panes[]"=w48:refnum<vi>[])  [unwired: 1 in, 2 out]
  n169 = property on="Camera Settings" class="Clust (strict)"("Val(Sgnl)"=w51) -> ()  [unwired: 2 in, 2 out]
  n170 = Index Array(array=w48) -> (element=w46:refnum<vi>)  [unwired: 1 in]
  n171 = control-ref of="Test Tree"() -> (w49:refnum<vi>)
  n172 = while {
    tunnel: w52 -> [w309]
    shift-right: [w308] -> _
    shift-left: w50 -> [w307]
    tunnel: [w306] -> _
    tunnel: w49 -> [w305]
    tunnel: w45 -> [w304]
    tunnel: w44 -> [w303]
    tunnel: w43 -> [_]
    tunnel: w39 -> [w302]
    i -> [w306]
    stop <- FALSE stop-if-true
    n173 = event shown="[0] Timeout" {
      selector: w303 -> [_ _ _ _ _ _ _ _ _ _ _ _ _ _ _ _ _]
      dyn-events: [_ _ _ _ _ _ _ _ _ _ _ _ _ w547 _ _ _] -> _
      timeout: u32 60 ("milliseconds to wait") -> [_ _ _ _ _ _ _ _ _ _ _ _ _ _ _ _ _]
      tunnel: w305 -> [w321 _ _ _ _ _ _ _ _ _ _ _ _ _ _ _ _]
      tunnel: "Test Tree" -> [_ _ _ _ _ _ _ _ w516 w524 w526 w530 w538 _ _ _ _]
      tunnel: w309 -> [_ w343 _ _ _ _ w480 w510 _ _ _ _ _ _ _ _ _]
      tunnel: [w317 w342 w441 w446 w454 w466 w479 w503 w515 w522 w525 w529 w537 w549 w563 w564 w574] -> w308
      tunnel: w307 -> [w317 w342 w441 w446 w454 w466 w478 w503 w515 w522 w525 w529 w537 w549 w563 w564 w574]
      tunnel: w304 -> [_ _ _ _ _ _ _ _ _ _ _ _ _ w550 _ w567 _]
      tunnel: w302 -> [_ _ _ _ _ _ _ _ _ _ _ _ _ w545 _ _ _]
      event Timeout {
        n174 = event-data() -> ()  [unwired: 1 in, 1 out]
        n175 = local read "Mode"() -> (w320:T6)
        n176 = Index Array(array=T30 [{"Operation"=enum."Clear", "Color Box"=14013909}, {"Operation"=enum."Clear", "Color Box"=14013909}, {"Operation"=enum."Clear", "Color Box"=14013909}, {"Operation"=enum."Clear", "Color Box"=14013909}, {"Operation"=enum."Update", "Color Box"=14013909}, {"Operation"=enum."Update", "Color Box"=16777215}, {"Operation"=enum."Clear", "Color Box"=14013909}, {"Operation"=enum."Clear", "Color Box"=14013909}, {"Operation"=enum."Clear", "Color Box"=14013909}], index=w320) -> (element=w315:T34)
        n177 = Unbundle(w315) -> ("Operation"=w314:enum16{"Update", "Clear"}, "Color Box"=w313:u32)
        n178 = call <vilib>:"NT Read String.vi"("Name"="TestMode/TestName") -> ("String"=w324:string)  [unwired: 9 in, 1 out]
        n179 = case shown="\"Variables\"" "Dashboard Tab" {
          tunnel: w321 -> [_ w332 _]
          tunnel: "/TestMode/Automatic/" ("Name Pattern") -> [_ w331 _]
          tunnel: w314 -> [_ w330 _]
          tunnel: [_ _ w334] -> _
          tunnel: w313 -> [_ w326 _]
          frame "Calibrations", Default {
          }
          frame "Test" {
            w329 = -2 ("Active Item:Row Number")
            n180 = call <vilib>:"NT Read and Format Entries as Tree.vi"("Operation"=w330, "Name Pattern"=w331, "Tree Refnum"=w332) -> ()  [unwired: 7 in, 2 out]
            n181 = property on="Test Tree" class="Tree (strict)"("Active Item Row Number"=w329, "ActiveColNum"=w329, "CellBG"=w326, "Active Item Row Number"=-1 ("Active Item:Row Number"), "CellBG"=u32 5789784 ("Color Box")) -> ()  [unwired: 2 in, 2 out]
          }
          frame "Variables" {
            n182 = control-ref of="Tree"() -> (w333:refnum<vi>)
            n183 = call <vilib>:"NT Read and Format Entries as Tree.vi"("Tree Refnum"=w333) -> ("Formatted Strings"=w334:cluster{"Name":string, "Value":string}[])  [unwired: 9 in, 1 out]
          }
        }
        n184 = case shown="Default" w324 {
          tunnel: "TestMode/TestProgress" ("Name") -> [w336 _]
          tunnel: "TestMode/TestProgressText" ("Name") -> [w335 _]
          frame Default {
            n185 = call <vilib>:"NT Read Number.vi"("Name"=w336) -> ("Numeric"=w337:dbl)  [unwired: 9 in, 1 out]
            n186 = call <vilib>:"NT Read String.vi"("Name"=w335) -> ("String"=w338:string)  [unwired: 9 in, 1 out]
            n187 = Bundle("Numeric"=w337, "String"=w338) -> (→"Progress":cluster{"Numeric":dbl, "String":string})  [unwired: 1 in]
          }
          frame "" {
            n188 = property on="Progress" class="Clust (strict)"("Visible"=FALSE) -> ()  [unwired: 2 in, 2 out]
            n189 = local write "Test Name"(u16 0) -> ()
          }
        }
      }
      event "Test Tree": Value Change {
        # "Show appropriate\ncontrols"
        n190 = event-data() -> ("CtlRef"=w346:refnum<vi>, "NewVal"=w344:string)  [unwired: 1 in]
        n191 = call <vilib>:"WPI_UtilitiesGetTreeIOName.vi"("NewVal"=w344, "TreeControl in"=w346) -> ("I/O Name"=w347:string)  [unwired: 9 in]
        n192 = case shown="\"Camera\"" w347 {
          selector: w347 -> [_ w354 _ w372 w381 _]
          tunnel: w344 -> [_ _ w369 w371 _ w388]
          tunnel: w343 -> [_ _ _ _ _ w387]
          frame Default {
            w349 = FALSE ("Visible")
            w348 = FALSE ("Visible")
            n193 = property on="Motor" class="Clust (strict)"("Visible"=w348) -> ()  [unwired: 2 in, 2 out]
            n194 = property on="Test Ring" class="Ring (strict)"("Visible"=w348) -> ()  [unwired: 2 in, 2 out]
            n195 = property on="Rev/Fwd" class="Clust (strict)"("Visible"=w349) -> ()  [unwired: 2 in, 2 out]
            n196 = property on="On/Off" class="Bool (strict)"("Visible"=w349) -> ()  [unwired: 2 in, 2 out]
            n197 = property on="Test Slider" class="Slide (strict)"("Visible"=w349) -> ()  [unwired: 2 in, 2 out]
          }
          frame "Motor", "PWM" {
            w355 = FALSE ("Visible")
            n198 = case shown="\"Motor\", Default" w354 {
              tunnel: [1.0 ("Value") -1.0 ("Value")] -> w353
              tunnel: [255.0 ("Value") 1.0 ("Value")] -> w352
              tunnel: [128.0 ("Value") 0.0 ("Value")] -> w351
              tunnel: [64.0 ("Value") 0.5 ("Value")] -> w350
              frame "PWM" {
              }
              frame "Motor", Default {
              }
            }
            n199 = property on="Motor" class="Clust (strict)"("Visible"=TRUE) -> ()  [unwired: 2 in, 2 out]
            n200 = property on="Value" class="Slide (strict)"("Value"=w351, "Scale.Minimum"=w353, "Scale.Maximum"=w352, "Scale.Increment"=w350) -> ()  [unwired: 2 in, 2 out]
            n201 = property on="On/Off" class="Bool (strict)"("Visible"=w355) -> ()  [unwired: 2 in, 2 out]
            n202 = property on="Test Slider" class="Slide (strict)"("Visible"=w355) -> ()  [unwired: 2 in, 2 out]
            n203 = property on="Test Ring" class="Ring (strict)"("Visible"=w355) -> ()  [unwired: 2 in, 2 out]
            n204 = property on="Rev/Fwd" class="Clust (strict)"("Visible"=w355) -> ()  [unwired: 2 in, 2 out]
          }
          frame "Servo" {
            w367 = FALSE ("Visible")
            n205 = call <vilib>:"NT Read Number.vi"("Name"=w369) -> ("Numeric"=w368:dbl)  [unwired: 9 in, 1 out]
            n206 = property on="Test Slider" class="Slide (strict)"("Visible"=TRUE, "Scale.Maximum"=170.0 ("Scale.Range:Maximum")) -> ()  [unwired: 2 in, 2 out]
            n207 = local write "Test Slider"(w368) -> ()
            n208 = property on="Motor" class="Clust (strict)"("Visible"=w367) -> ()  [unwired: 2 in, 2 out]
            n209 = property on="Rev/Fwd" class="Clust (strict)"("Visible"=w367) -> ()  [unwired: 2 in, 2 out]
            n210 = property on="On/Off" class="Bool (strict)"("Visible"=w367) -> ()  [unwired: 2 in, 2 out]
            n211 = property on="Test Ring" class="Ring (strict)"("Visible"=w367) -> ()  [unwired: 2 in, 2 out]
          }
          frame "Relay", "Solenoid" {
            w370 = FALSE ("Visible")
            n212 = property on="Motor" class="Clust (strict)"("Visible"=w370) -> ()  [unwired: 2 in, 2 out]
            n213 = property on="Test Slider" class="Slide (strict)"("Visible"=w370) -> ()  [unwired: 2 in, 2 out]
            n214 = Search and Replace String(input string=w371, search string="/Value  **", replace string="/Direction") -> (result string=w377:string)  [unwired: 5 in, 3 out]
            n215 = property on="Test Ring" class="Ring (strict)"("Visible"=w370) -> ()  [unwired: 2 in, 2 out]
            n216 = call <vilib>:"NT Read String.vi"("Name"=w377) -> ("String"=w375:string)  [unwired: 9 in, 1 out]
            n217 = Equal?(x="Both directions", y=w375) -> (x = y?=w373:bool)
            n218 = Not(x=w373) -> (.not. x?=w374:bool)
            n219 = property on="Rev/Fwd" class="Clust (strict)"("Visible"=w373) -> ()  [unwired: 2 in, 2 out]
            n220 = property on="On/Off" class="Bool (strict)"("Visible"=w374, "Caption.Text"=w372) -> ()  [unwired: 2 in, 2 out]
          }
          frame "Compressor", "Digital Out" {
            w380 = FALSE ("Visible")
            # "Get direction and finish"
            n221 = property on="Motor" class="Clust (strict)"("Visible"=w380) -> ()  [unwired: 2 in, 2 out]
            n222 = property on="Test Slider" class="Slide (strict)"("Visible"=w380) -> ()  [unwired: 2 in, 2 out]
            n223 = property on="Test Ring" class="Ring (strict)"("Visible"=w380) -> ()  [unwired: 2 in, 2 out]
            n224 = property on="On/Off" class="Bool (strict)"("Visible"=TRUE, "Caption.Text"=w381) -> ()  [unwired: 2 in, 2 out]
            n225 = property on="Rev/Fwd" class="Clust (strict)"("Visible"=FALSE) -> ()  [unwired: 2 in, 2 out]
          }
          frame "Camera" {
            n226 = call <vilib>:"Get Last Path Segment.vi"("String in"=w388) -> ("String out"=w389:string)  [unwired: 10 in]
            n227 = property on="On/Off" class="Bool (strict)"("Visible"=FALSE) -> ()  [unwired: 2 in, 2 out]
            n228 = property on="Motor" class="Clust (strict)"("Visible"=FALSE) -> ()  [unwired: 2 in, 2 out]
            n229 = property on="Rev/Fwd" class="Clust (strict)"("Visible"=FALSE) -> ()  [unwired: 2 in, 2 out]
            n230 = case shown="\"White Balance  **\"" w389 {
              tunnel: w388 -> [w395 w404 w413 w422 w431 _ w437]
              tunnel: w387 -> [w393 w401 w410 w419 w428 _ _]
              frame "Size  **" {
                n231 = Index Array(array=w393) -> (element=w392:cluster{string[]})  [unwired: 1 in]
                n232 = call <vilib>:"NT Read String.vi"("Name"=w395) -> ("String"=w394:string)  [unwired: 9 in, 1 out]
                n233 = Unbundle(w392) -> (w390:string[])
                n234 = Match First String(2:w390, 3:w394) -> (0:w391:i32)  [unwired: 1 out]
                n235 = property on="Test Ring" class="Ring (strict)"("Value"=w391, "Strings []"=w390) -> ()  [unwired: 2 in, 2 out]
                n236 = property on="Test Ring" class="Ring (strict)"("Visible"=TRUE) -> ()  [unwired: 2 in, 2 out]
                n237 = property on="Test Slider" class="Slide (strict)"("Visible"=FALSE) -> ()  [unwired: 2 in, 2 out]
              }
              frame "White Balance  **" {
                n238 = Index Array(array=w401, index=1) -> (element=w402:cluster{string[]})
                n239 = call <vilib>:"NT Read String.vi"("Name"=w404) -> ("String"=w403:string)  [unwired: 9 in, 1 out]
                n240 = Unbundle(w402) -> (w399:string[])
                n241 = Match First String(2:w399, 3:w403) -> (0:w398:i32)  [unwired: 1 out]
                n242 = property on="Test Ring" class="Ring (strict)"("Value"=w398, "Strings []"=w399) -> ()  [unwired: 2 in, 2 out]
                n243 = property on="Test Ring" class="Ring (strict)"("Visible"=TRUE) -> ()  [unwired: 2 in, 2 out]
                n244 = property on="Test Slider" class="Slide (strict)"("Visible"=FALSE) -> ()  [unwired: 2 in, 2 out]
              }
              frame "Exposure  **" {
                n245 = Index Array(array=w410, index=2) -> (element=w411:cluster{string[]})
                n246 = call <vilib>:"NT Read String.vi"("Name"=w413) -> ("String"=w412:string)  [unwired: 9 in, 1 out]
                n247 = Unbundle(w411) -> (w407:string[])
                n248 = Match First String(2:w407, 3:w412) -> (0:w408:i32)  [unwired: 1 out]
                n249 = property on="Test Ring" class="Ring (strict)"("Value"=w408, "Strings []"=w407) -> ()  [unwired: 2 in, 2 out]
                n250 = property on="Test Ring" class="Ring (strict)"("Visible"=TRUE) -> ()  [unwired: 2 in, 2 out]
                n251 = property on="Test Slider" class="Slide (strict)"("Visible"=FALSE) -> ()  [unwired: 2 in, 2 out]
              }
              frame "Exposure Priority  **" {
                n252 = Index Array(array=w419, index=3) -> (element=w420:cluster{string[]})
                n253 = call <vilib>:"NT Read String.vi"("Name"=w422) -> ("String"=w421:string)  [unwired: 9 in, 1 out]
                n254 = Unbundle(w420) -> (w416:string[])
                n255 = Match First String(2:w416, 3:w421) -> (0:w417:i32)  [unwired: 1 out]
                n256 = property on="Test Ring" class="Ring (strict)"("Value"=w417, "Strings []"=w416) -> ()  [unwired: 2 in, 2 out]
                n257 = property on="Test Ring" class="Ring (strict)"("Visible"=TRUE) -> ()  [unwired: 2 in, 2 out]
                n258 = property on="Test Slider" class="Slide (strict)"("Visible"=FALSE) -> ()  [unwired: 2 in, 2 out]
              }
              frame "Color Enable  **" {
                n259 = Index Array(array=w428, index=4) -> (element=w429:cluster{string[]})
                n260 = call <vilib>:"NT Read String.vi"("Name"=w431) -> ("String"=w430:string)  [unwired: 9 in, 1 out]
                n261 = Unbundle(w429) -> (w425:string[])
                n262 = Match First String(2:w425, 3:w430) -> (0:w426:i32)  [unwired: 1 out]
                n263 = property on="Test Ring" class="Ring (strict)"("Value"=w426, "Strings []"=w425) -> ()  [unwired: 2 in, 2 out]
                n264 = property on="Test Ring" class="Ring (strict)"("Visible"=TRUE) -> ()  [unwired: 2 in, 2 out]
                n265 = property on="Test Slider" class="Slide (strict)"("Visible"=FALSE) -> ()  [unwired: 2 in, 2 out]
              }
              frame Default {
                n266 = property on="Test Ring" class="Ring (strict)"("Visible"=FALSE) -> ()  [unwired: 2 in, 2 out]
                n267 = property on="Test Slider" class="Slide (strict)"("Visible"=FALSE) -> ()  [unwired: 2 in, 2 out]
              }
              frame "Brightness  **", "Color Level  **", "Compression  **", "FPS  **", "Sharpness  **" {
                n268 = call <vilib>:"NT Read Number.vi"("Name"=w437) -> ("Numeric"=w436:dbl)  [unwired: 9 in, 1 out]
                n269 = local write "Test Slider"(w436) -> ()
                n270 = property on="Test Slider" class="Slide (strict)"("Visible"=TRUE, "Scale.Maximum"=100.0 ("Scale.Range:Maximum")) -> ()  [unwired: 2 in, 2 out]
                n271 = property on="Test Ring" class="Ring (strict)"("Visible"=FALSE) -> ()  [unwired: 2 in, 2 out]
              }
            }
          }
        }
        n272 = property on="Progress" class="Clust (strict)"("Visible"=FALSE) -> ()  [unwired: 2 in, 2 out]
      }
      event "Test Name": Mouse Enter {
        # "Populate the ring with the list of tests"
        n273 = event-data() -> ()  [unwired: 1 in, 1 out]
        n274 = call <vilib>:"NT Read String Array.vi"("Name"="TestMode/TestList") -> ("String Array"=w445:string[])  [unwired: 9 in, 1 out]
        n275 = Build Array (concatenate)("Select the test to run...", w445) -> (w444:string[])
        n276 = property on="Test Name" class="Ring (strict)"("Strings []"=w444) -> ()  [unwired: 2 in, 2 out]
      }
      event "Test Name": Value Change {
        w447 = FALSE ("Visible")
        # "Tell the robot the test name to run"
        n277 = event-data() -> ("NewVal"=w451:u16)  [unwired: 1 in]
        n278 = property on="Test Name" class="Ring (strict)"() -> ("Strings []"=w452:string[])  [unwired: 2 in, 2 out]
        n279 = local write "Progress"(T8 {"Test Progress"=0, "Test Progress Text"=""} ("Progress")) -> ()
        n280 = Index Array(array=w452, index=w451) -> (element=w450:string)
        n281 = call <vilib>:"NT Write String.vi"("String"=w450, "Name"="TestMode/TestName") -> ()  [unwired: 9 in, 1 out]
        n282 = property on="Progress" class="Clust (strict)"("Visible"=TRUE) -> ()  [unwired: 2 in, 2 out]
        n283 = property on="Motor" class="Clust (strict)"("Visible"=w447) -> ()  [unwired: 2 in, 2 out]
        n284 = property on="Test Slider" class="Slide (strict)"("Visible"=w447) -> ()  [unwired: 2 in, 2 out]
        n285 = property on="On/Off" class="Bool (strict)"("Visible"=w447) -> ()  [unwired: 2 in, 2 out]
        n286 = property on="Rev/Fwd" class="Clust (strict)"("Visible"=w447) -> ()  [unwired: 2 in, 2 out]
        n287 = property on="Test Ring" class="Ring (strict)"("Visible"=w447) -> ()  [unwired: 2 in, 2 out]
      }
      event "Listbox": Double Click {
        # "Shift clears all"
        # "Update symbols on the listbox"
        n288 = event-data() -> ("PlatMods.Shift"=w455:bool, "Row"=w457:i32)  [unwired: 1 in]
        n289 = case shown="True" w455 {
          tunnel: w457 -> [w461 _]
          tunnel: 1 -> [w460 _]
          frame False {
            n290 = property on="Listbox" class="LstBox (strict)"() -> ("Item Symbols"=w459:i32[])  [unwired: 2 in, 2 out]
            n291 = Replace Array Subset(array=w459, new element=w460, index=w461) -> (w458:i32[])
            n292 = property on="Listbox" class="LstBox (strict)"("Item Symbols"=w458) -> ()  [unwired: 2 in, 2 out]
          }
          frame True {
            w462 = 0 ("Top Row")
            n293 = property on="Listbox" class="LstBox (strict)"() -> ("Number of Rows"=w464:u32)  [unwired: 2 in, 2 out]
            n294 = Initialize Array(0, w464) -> (w463:i32[])
            n295 = property on="Listbox" class="LstBox (strict)"("Top Row"=w462, "Value"=w462, "Item Symbols"=w463) -> ()  [unwired: 2 in, 2 out]
          }
        }
      }
      event "Listbox": Key Down {
        # "Update symbols on the listbox\nLeft and right keys check and uncheck"
        n296 = event-data() -> ("VKey"=w468:T31)  [unwired: 1 in]
        n297 = case shown="\"Left\", \"Right\"" w468 {
          selector: w468 -> [w473 _]
          tunnel: eventvkey."Left" ("VKey") -> [w471 _]
          frame "Left", "Right" {
            n298 = Equal?(x=w471, y=w473) -> (x = y?=w472:bool)
            n299 = Select(t=0, s=w472, f=1) -> (s? t:f=w474:i32)
            n300 = property on="Listbox" class="LstBox (strict)"() -> ("Item Symbols"=w477:i32[])  [unwired: 2 in, 2 out]
            n301 = Replace Array Subset(array=w477, new element=w474, index="Listbox") -> (w476:i32[])
            n302 = property on="Listbox" class="LstBox (strict)"("Item Symbols"=w476) -> ()  [unwired: 2 in, 2 out]
          }
          frame Default {
          }
        }
      }
      event "DB Camera Config": Value Change {
        # "Show or hide the cluster of controls, store in ini file"
        n303 = event-data() -> ("NewVal"=w481:bool)  [unwired: 1 in]
        n304 = case shown="False" w481 {
          tunnel: w480 -> [w490 _]
          tunnel: [w483 w501] -> w479
          tunnel: w478 -> [w482 w501]
          frame False {
            w497 = "Camera"
            w500 = FALSE ("Visible")
            n305 = local read "Camera Settings"() -> (w489:T2)
            n306 = Index Array(array=w490) -> (element=w493:cluster{string[]})  [unwired: 1 in]
            n307 = Unbundle(w489) -> ("Frame Rate"=w488:i32, "Compression"=w487:i32, "Size"=w491:u16)
            n308 = Unbundle(w493) -> (w492:string[])
            n309 = Index Array(array=w492, index=w491) -> (element=w486:string)
            n310 = call-poly <vilib>:"Write Key.vi"("section"=w497, "value"=w486, "key"="Size", "refnum"=w482) -> ("refnum out"=w499:T29)  [unwired: 2 in, 5 out]
            n311 = call-poly <vilib>:"Write Key.vi"("section"=w497, "value"=w488, "key"="FrameRate", "refnum"=w499) -> ("refnum out"=w498:T29)  [unwired: 1 in, 6 out]
            n312 = property on="Camera Settings" class="Clust (strict)"("Visible"=w500) -> ()  [unwired: 2 in, 2 out]
            n313 = local write "DB Camera Config"(w500) -> ()
            n314 = call-poly <vilib>:"Write Key.vi"("section"=w497, "value"=w487, "key"="Compression", "refnum"=w498) -> ("refnum out"=w484:T29)  [unwired: 1 in, 6 out]
            n315 = call <vilib>:"Close Config Data.vi"("refnum"=w484) -> ("file path"=w485:path)  [unwired: 2 in, 8 out]
            n316 = call <vilib>:"Open Config Data.vi"("configuration file path"=w485) -> ("refnum"=w483:T29)  [unwired: 8 in, 2 out]
          }
          frame True {
            n317 = property on="Camera Settings" class="Clust (strict)"("Visible"=TRUE) -> ()  [unwired: 2 in, 2 out]
          }
        }
      }
      event "Camera Settings": Value Change {
        # "Update summary string when any elements of DB camera change"
        n318 = event-data() -> ("NewVal"=w514:T2)  [unwired: 1 in]
        n319 = Index Array(array=w510) -> (element=w509:cluster{string[]})  [unwired: 1 in]
        n320 = Unbundle(w514) -> ("Frame Rate"=w505:i32, "Compression"=w504:i32, "Size"=w507:u16)
        n321 = Unbundle(w509) -> (w508:string[])
        n322 = Index Array(array=w508, index=w507) -> (element=w506:string)
        n323 = Format Into String(format string="%s   %dfps   %d%%", w506, w505, w504) -> (resulting string=w511:string)  [unwired: 2 in, 1 out]
        n324 = Build Array(w511) -> (w512:string[])
        n325 = property on="DB Camera Config" class="Bool (strict)"("Strings [4]"=w512) -> ()  [unwired: 2 in, 2 out]
      }
      event "Motor.Enable": Value Change {
        # "When the test mode otor enable helper is set, update that\ntree row item's value"
        n326 = event-data() -> ("NewVal"=w520:bool)  [unwired: 1 in]
        n327 = Unbundle("Motor") -> ("Value"=w519:dbl)  [unwired: 1 out]
        n328 = Select(t=w519, s=w520, f=0.0) -> (s? t:f=w517:dbl)
        n329 = call <vilib>:"NT Write Number.vi"("Numeric"=w517, "Name"=w516) -> ()  [unwired: 9 in, 1 out]
      }
      event "Test Slider": Value Change {
        # "When the test mode slider helper is set, update that\ntree row item's value"
        n330 = event-data() -> ("NewVal"=w523:dbl)  [unwired: 1 in]
        n331 = call <vilib>:"NT Write Number.vi"("Numeric"=w523, "Name"=w524) -> ()  [unwired: 9 in, 1 out]
      }
      event "On/Off": Value Change {
        # "When the test mode on/off helper value is set, update that\ntree row item's value"
        n332 = event-data() -> ("NewVal"=w528:bool)  [unwired: 1 in]
        n333 = Boolean To (0,1)(Boolean=w528) -> (0, 1=w527:i16)
        n334 = call <vilib>:"NT Write Number.vi"("Numeric"=w527, "Name"=w526) -> ()  [unwired: 9 in, 1 out]
      }
      event "Rev/Fwd": Value Change {
        # "When the test mode helper value for relays is set, update that\ntree row item's value"
        n335 = event-data() -> ("NewVal.Forward"=w536:bool, "NewVal.Reverse"=w535:bool)  [unwired: 1 in]
        n336 = Boolean To (0,1)(Boolean=w536) -> (0, 1=w532:i16)
        n337 = Boolean To (0,1)(Boolean=w535) -> (0, 1=w534:i16)
        n338 = Negate(x=w534) -> (-x=w533:i16)
        n339 = Add(x=w532, y=w533) -> (x+y=w531:i16)
        n340 = call <vilib>:"NT Write Number.vi"("Numeric"=w531, "Name"=w530) -> ()  [unwired: 9 in, 1 out]
      }
      event "Test Ring": Value Change {
        # "When a test mode helper value is selected from the ring,\nset the tree item's variable to the string value"
        n341 = event-data() -> ("NewVal"=w540:u16)  [unwired: 1 in]
        n342 = property on="Test Ring" class="Ring (strict)"() -> ("Strings []"=w541:string[])  [unwired: 2 in, 2 out]
        n343 = Index Array(array=w541, index=w540) -> (element=w539:string)
        n344 = call <vilib>:"NT Write String.vi"("String"=w539, "Name"=w538) -> ()  [unwired: 9 in, 1 out]
      }
      event "Rec Mode": Value Change {
        # "Update globals for recording mode and path to read log from.\nClear when logging and let NetworkTables set path for vision to\nuse."
        n345 = event-data() -> ("NewVal"=w551:enum32{"Stop", "Record", "Playback"})  [unwired: 1 in]
        n346 = global write "WPI_DashboardLogging Global.vi" "Logging Filename"(path "") -> ()
        n347 = case shown="\"Playback\"" w551 {
          tunnel: w550 -> [_ w553 w561]
          tunnel: [_ _ w560] -> w547
          tunnel: [_ _ w559] -> _
          tunnel: w545 -> [_ _ w557]
          tunnel: cluster{i32, i32} {-250, 170} -> [_ _ w556]
          tunnel: [_ _ T32 {"Image Size"=TRUE, "Image Type"=TRUE, "Pixel Value"=TRUE, "ROI Information"=TRUE, "Zoom Factor"=FALSE} ("Image Information Shown:All Elements")] -> w543
          tunnel: [_ _ TRUE ("Zoom Factor")] -> w542
          frame Default {
          }
          frame "Stop", "Record" {
            # "Place Window too"
            n348 = invoke class="VI" method="FP.Close"(reference=w553) -> (reference out=w552:refnum<vi>)  [unwired: 2 in, 2 out]
            n349 = invoke class="VI" method="Abort VI"(reference=w552) -> ()  [unwired: 2 in, 3 out]
          }
          frame "Playback" {
            n350 = call "Open Playback Panel.vi"("Offset"=w556, "DB VI Ref"=w557, "Playback in"=w561) -> ("Playback out"=w558:refnum<vi>)  [unwired: 8 in]
            n351 = register-events(w558) -> (reference out=w560:refnum<event-registration>, error out=w559:errorcluster)  [unwired: 2 in]
          }
        }
        n352 = global write "WPI_DashboardLogging Global.vi" "Recording"(w551) -> ()
        n353 = property on="Camera Image" class="ImageControl"("Image Information Shown"=w543, "Image Information Visible"=w542) -> ()  [unwired: 2 in, 2 out]
        n354 = call <vilib>:"WPI_DashboardNT Log FieldName Cache.vi"("Operation"=enum16{"Lookup/Add", "Index", "Clear"}."Clear") -> ()  [unwired: 8 in, 3 out]
      }
      event Panel Close {
        w562 = enum32{"Stop", "Record", "Playback"}."Stop" ("Rec Mode")
        # "Playback window has been closed, abort"
        n355 = event-data() -> ()  [unwired: 1 in, 4 out]
        n356 = local write "Rec Mode"(w562) -> ()
        n357 = global write "WPI_DashboardLogging Global.vi" "Recording"(w562) -> ()
      }
      event Panel Close {
        # "Abort playback window and ourself"
        n358 = event-data() -> ()  [unwired: 1 in, 4 out]
        n359 = invoke class="VI" method="FP.Close"(reference=w567) -> (reference out=w566:refnum<vi>)  [unwired: 2 in, 2 out]
        n360 = invoke class="VI" method="Abort VI"(reference=w566) -> (error out=w565:errorcluster)  [unwired: 2 in, 2 out]
        n361 = invoke class="VI" method="Abort VI"(error in=w565) -> ()  [unwired: 2 in, 3 out]
      }
      event "Vision": Value Change {
        # "Enable/Disable Compression slider.\nHW USB is hard-coded into the camera"
        n362 = event-data() -> ("NewVal"=w573:u16)  [unwired: 1 in]
        n363 = Equal?(x=w573, y=u32 2 ("milliseconds to wait")) -> (x = y?=w571:bool)
        n364 = Select(t=T33."Disabled and Grayed Out" ("Disabled"), s=w571, f=T33."Enabled" ("Disabled")) -> (s? t:f=w568:T33)
        n365 = property on="Compression" class="Slide (strict)"("DisabledEnum"=w568) -> ()  [unwired: 2 in, 2 out]
      }
    }
  }
  n366 = while {
    tunnel: w46 -> [w576]
    i -> [w579]
    stop <- FALSE stop-if-true
    n367 = Wait (ms)(milliseconds to wait=u32 100) -> ()  [unwired: 1 out]
    n368 = case shown="\"Playback\"" "Rec Mode" {
      tunnel: w579 -> [_ _ w594]
      tunnel: [u32 2829099 ("Base Color") u32 11141120 ("Target Color") w583] -> w575
      frame "Stop", Default {
        # "Reset the color, extra updates don't cost much"
      }
      frame "Record" {
      }
      frame "Playback" {
        # "Playback"
        n369 = Quotient & Remainder(x=w594, y=u32 50 ("milliseconds to wait")) -> (x-y*floor(x/y)=w590:u32)  [unwired: 1 out]
        n370 = Divide(x=w590, y=u32 50 ("milliseconds to wait")) -> (x/y=w587:dbl)
        n371 = Multiply(x=6.283185307179586, y=w587) -> (x*y=w592:dbl)
        n372 = Sine(x=w592) -> (sin(x)=w591:dbl)
        n373 = Absolute Value(x=w591) -> (abs(x)=w584:dbl)
        n374 = call "Interpolate RGB Color.vi"("Proportion"=w584, "Target Color"=u32 30976, "Base Color"=u32 2829099) -> ("Result Color"=w583:u32)  [unwired: 8 in]
      }
    }
    n375 = property class="Pane"(reference=w576, "PaneColor"=w575) -> ()  [unwired: 1 in, 2 out]
  }
  n376 = TCP Create Listener(10:u16 1741 ("timeout ms (25000)")) -> (3:w10:refnum<k5>)  [unwired: 4 in, 2 out]
  n377 = while {
    tunnel: w10 -> [w596]
    stop <- FALSE stop-if-true
    n378 = TCP Wait On Listener(11:w596) -> (4:w595:refnum<k5>)  [unwired: 3 in, 4 out]
    n379 = local write "TCP"(w595) -> ()
  }
  n380 = property on="On/Off" class="Bool (strict)"("Visible"=w15) -> ()  [unwired: 2 in, 2 out]
  n381 = property on="Motor" class="Clust (strict)"("Visible"=w15) -> ()  [unwired: 2 in, 2 out]
  n382 = property on="Progress" class="Clust (strict)"("Visible"=w15) -> ()  [unwired: 2 in, 2 out]
  n383 = property on="Test Ring" class="Ring (strict)"("Visible"=w15) -> ()  [unwired: 2 in, 2 out]
  n384 = property on="Rev/Fwd" class="Clust (strict)"("Visible"=w15) -> ()  [unwired: 2 in, 2 out]
  n385 = property on="Camera Settings" class="Clust (strict)"("Visible"=w15) -> ()  [unwired: 2 in, 2 out]
  n386 = local write "DB Camera Config"(w15) -> ()
  n387 = global write "WPI_DashboardLogging Global.vi" "Recording"(w40) -> ()
  n388 = local write "Rec Mode"(w40) -> ()
  "GetIniState" <- enum16{"Waiting", "SwitchModeHappening"}."Waiting" ("GetIniState")
  "SetIniState" <- enum16{"Waiting", "SwitchModeHappening"}."Waiting" ("SetIniState")
  "Camera Mode" <- FALSE ("Camera Mode")
  "CameraSwitchModeState" <- enum16{"Waiting", "SwitchModeHappening"}."Waiting" ("CameraSwitchModeState")
  "OpenIniState" <- enum16{"Waiting", "SwitchModeHappening"}."Waiting" ("GetIniState")
  "FTP Result" <- u32 9868950 ("Color Box")
